vi "rszvl_core_global.vi"() -> ()   [LabVIEW 2014] (continued)
Repeated Capabilities"="", "Help"="This attribute returns the determined CREST factor (= ratio of peak power to average power) in dB.\n\nAvailable Repeated Capabilities:\nModifMinMaxAver: Min,Max,Aver\r\n\nRemote-control command(s):\nFETCh:BURSt:CRESt<[:AVERage] | :MAXimum|:MIMimum>?", "Flags"={"OPC Wait"=FALSE, "Dont check status"=FALSE, "*WAI"=FALSE}, "Check Status Callback"=""}, {"Level"=3, "Descriptive Name"="WLAN Fetch Rise Time", "Class Only"=FALSE, "Data Type"=1, "Access"=0, "Identifier"="RSZVL_ATTR_WLAN_FETC_TRIS", "Range Table"="", "Command"="FETC:BURS:TRIS:{ModifMinMaxAver}?", "Read Callback"="", "Write Callback"="", "Range Callback"="", "Check Callback"="", "Rngtable Callback"="", "Coerce Callback"="", "User Callback"="", "Supported Models"="", "Instrument Options"="", "Repeated Capabilities"="", "Restricted Repeated Capabilities"="", "Help"="This attribute returns the burst rise time in seconds.\n\nNote:\n(1) This attribute is valid only if standard IEEE 802.11b is selected.\n\nAvailable Repeated Capabilities:\nModifMinMaxAver: Min,Max,Aver\r\n\nRemote-control command(s):\nFETCh:BURSt:TRISe:<AVERage | MAXimum | MIMimum>?", "Flags"={"OPC Wait"=FALSE, "Dont check status"=FALSE, "*WAI"=FALSE}, "Check Status Callback"=""}, {"Level"=3, "Descriptive Name"="WLAN Fetch Fall Time", "Class Only"=FALSE, "Data Type"=1, "Access"=0, "Identifier"="RSZVL_ATTR_WLAN_FETC_TFAL", "Range Table"="", "Command"="FETC:BURS:TFAL:{ModifMinMaxAver}?", "Read Callback"="", "Write Callback"="", "Range Callback"="", "Check Callback"="", "Rngtable Callback"="", "Coerce Callback"="", "User Callback"="", "Supported Models"="", "Instrument Options"="", "Repeated Capabilities"="", "Restricted Repeated Capabilities"="", "Help"="This attribute returns the burst fall time in seconds.\n\nNote :\n(1) This attribute is available only for IEEE 802.11b standard.\n\nAvailable Repeated Capabilities:\nModifMinMaxAver: Min,Max,Aver\r\n\nRemote-control command(s):\nFETCh:BURSt:TFALl:<AVERage | MAXimum | MIMimum>?", "Flags"={"OPC Wait"=FALSE, "Dont check status"=FALSE, "*WAI"=FALSE}, "Check Status Callback"=""}, {"Level"=3, "Descriptive Name"="WLAN Fetch Frequency Error", "Class Only"=FALSE, "Data Type"=1, "Access"=0, "Identifier"="RSZVL_ATTR_WLAN_FETC_FERR", "Range Table"="", "Command"="FETC:BURS:FERR:{ModifMinMaxAver}?", "Read Callback"="", "Write Callback"="", "Range Callback"="", "Check Callback"="", "Rngtable Callback"="", "Coerce Callback"="", "User Callback"="", "Supported Models"="", "Instrument Options"="", "Repeated Capabilities"="", "Restricted Repeated Capabilities"="", "Help"="This attribute returns the measured frequency error in Hz.\n\nAvailable Repeated Capabilities:\nModifMinMaxAver: Min,Max,Aver\r\n\nRemote-control command(s):\nFETCh:BURSt:FERRor:<AVERage | MAXimum | MIMimum>?", "Flags"={"OPC Wait"=FALSE, "Dont check status"=FALSE, "*WAI"=FALSE}, "Check Status Callback"=""}, {"Level"=3, "Descriptive Name"="WLAN Fetch Symbol Error", "Class Only"=FALSE, "Data Type"=1, "Access"=0, "Identifier"="RSZVL_ATTR_WLAN_FETC_SYMB", "Range Table"="", "Command"="FETC:BURS:SYMB:{ModifMinMaxAver}?", "Read Callback"="", "Write Callback"="", "Range Callback"="", "Check Callback"="", "Rngtable Callback"="", "Coerce Callback"="", "User Callback"="", "Supported Models"="", "Instrument Options"="", "Repeated Capabilities"="", "Restricted Repeated Capabilities"="", "Help"="This attribute returns the number of symbols  that were outside the permissible demodulation\nrange within a burst.\n\nAvailable Repeated Capabilities:\nModifMinMaxAver: Min,Max,Aver\r\n\nRemote-control command(s):\nFETCh:BURSt:SYMBolerror:<AVERage | MAXimum | MIMimum>?", "Flags"={"OPC Wait"=FALSE, "Dont check status"=FALSE, "*WAI"=FALSE}, "Check Status Callback"=""}, {"Level"=3, "Descriptive Name"="WLAN Fetch IQ Offset Error", "Class Only"=FALSE, "Data Type"=1, "Access"=0, "Identifier"="RSZVL_ATTR_WLAN_FETC_IQOF", "Range Table"="", "Command"="FETC:BURS:IQOF:{ModifMinMaxAver}?", "Read Callback"="", "Write Callback"="", "Range Callback"="", "Check Callback"="", "Rngtable Callback"="", "Coerce Callback"="", "User Callback"="", "Supported Models"="", "Instrument Options"="", "Repeated Capabilities"="", "Restricted Repeated Capabilities"="", "Help"="This attribute returns the measured IQ offset errors in dB.\n\nAvailable Repeated Capabilities:\nModifMinMaxAver: Min,Max,Aver\r\n\nRemote-control command(s):\nFETCh:BURSt:IQOFfset:<AVERage | MAXimum | MIMimum>?", "Flags"={"OPC Wait"=FALSE, "Dont check status"=FALSE, "*WAI"=FALSE}, "Check Status Callback"=""}, {"Level"=3, "Descriptive Name"="WLAN Fetch IQ Imbalance Error", "Class Only"=FALSE, "Data Type"=1, "Access"=0, "Identifier"="RSZVL_ATTR_WLAN_FETC_GIMB", "Range Table"="", "Command"="FETC:BURS:GIMB:{ModifMinMaxAver}?", "Read Callback"="", "Write Callback"="", "Range Callback"="", "Check Callback"="", "Rngtable Callback"="", "Coerce Callback"="", "User Callback"="", "Supported Models"="", "Instrument Options"="", "Repeated Capabilities"="", "Restricted Repeated Capabilities"="", "Help"="This attribute returns the measured IQ imbalance errors in dB.\n\nAvailable Repeated Capabilities:\nModifMinMaxAver: Min,Max,Aver\r\n\nRemote-control command(s):\nFETCh:BURSt:GIMBalance:<AVERage | MAXimum | MIMimum>?", "Flags"={"OPC Wait"=FALSE, "Dont check status"=FALSE, "*WAI"=FALSE}, "Check Status Callback"=""}, {"Level"=3, "Descriptive Name"="WLAN Fetch Quadrature Error", "Class Only"=FALSE, "Data Type"=1, "Access"=0, "Identifier"="RSZVL_ATTR_WLAN_FETC_QUAD", "Range Table"="", "Command"="FETC:BURS:QUAD:{ModifMinMaxAver}?", "Read Callback"="", "Write Callback"="", "Range Callback"="", "Check Callback"="", "Rngtable Callback"="", "Coerce Callback"="", "User Callback"="", "Supported Models"="", "Instrument Options"="", "Repeated Capabilities"="", "Restricted Repeated Capabilities"="", "Help"="This attribute returns the accuracy in terms of the phase error of symbols within a burst.\nIt returns the angle error recorded for a symbol during the measurement.\n\nAvailable Repeated Capabilities:\nModifMinMaxAver: Min,Max,Aver\r\n\nRemote-control command(s):\nFETCh:BURSt:QUADoffset:<AVERage | MAXimum | MIMimum>?", "Flags"={"OPC Wait"=FALSE, "Dont check status"=FALSE, "*WAI"=FALSE}, "Check Status Callback"=""}, {"Level"=3, "Descriptive Name"="WLAN Fetch EVM", "Class Only"=FALSE, "Data Type"=1, "Access"=0, "Identifier"="RSZVL_ATTR_WLAN_FETC_EVM", "Range Table"="", "Command"="FETC:BURS:EVM:{ModifMinMaxAver}?", "Read Callback"="", "Write Callback"="", "Range Callback"="", "Check Callback"="", "Rngtable Callback"="", "Coerce Callback"="", "User Callback"="", "Supported Models"="", "Instrument Options"="", "Repeated Capabilities"="", "Restricted Repeated Capabilities"="", "Help"="This attribute returns the error vector magnitude measurement results summary in dB for the IEEE 802.11b standard. This result is the value before filtering.\n\nNote :\n(1) This attribute is available only for IEEE 802.11b standard.\n\nAvailable Repeated Capabilities:\nModifMinMaxAver: Min,Max,Aver\r\n\nRemote-control command(s):\nFETCh:BURSt:EVM:[IEEE]:<AVERage | MAXimum | MIMimum>?", "Flags"={"OPC Wait"=FALSE, "Dont check status"=FALSE, "*WAI"=FALSE}, "Check Status Callback"=""}, {"Level"=3, "Descriptive Name"="WLAN Fetch Filtered EVM", "Class Only"=FALSE, "Data Type"=1, "Access"=0, "Identifier"="RSZVL_ATTR_WLAN_FETC_EVM_DIR", "Range Table"="", "Command"="FETC:BURS:EVM:DIR:{ModifMinMaxAver}?", "Read Callback"="", "Write Callback"="", "Range Callback"="", "Check Callback"="", "Rngtable Callback"="", "Coerce Callback"="", "User Callback"="", "Supported Models"="", "Instrument Options"="", "Repeated Capabilities"="", "Restricted Repeated Capabilities"="", "Help"="This attribute returns the error vector magnitude measurement results summary in dB for the IEEE 802.11b standard. This result is the value after filtering.\n\nNote :\n(1) This attribute is available only for IEEE 802.11b standard.\n\nAvailable Repeated Capabilities:\nModifMinMaxAver: Min,Max,Aver\r\n\nRemote-control command(s):\nFETCh:BURSt:EVM:DIRect:<AVERage | MAXimum | MIMimum>?", "Flags"={"OPC Wait"=FALSE, "Dont check status"=FALSE, "*WAI"=FALSE}, "Check Status Callback"=""}, {"Level"=3, "Descriptive Name"="WLAN Fetch EVM All Carriers", "Class Only"=FALSE, "Data Type"=1, "Access"=0, "Identifier"="RSZVL_ATTR_WLAN_FETC_EVM_ALL", "Range Table"="", "Command"="FETC:BURS:EVM:ALL:{ModifMinMaxAver}?", "Read Callback"="", "Write Callback"="", "Range Callback"="", "Check Callback"="", "Rngtable Callback"="", "Coerce Callback"="", "User Callback"="", "Supported Models"="", "Instrument Options"="", "Repeated Capabilities"="", "Restricted Repeated Capabilities"="", "Help"="This attribute returns the error vector magnitude measurement results summary in dB. This is a combined figure that represents the pilot, data and the free carrier.\n\nAvailable Repeated Capabilities:\nModifMinMaxAver: Min,Max,Aver\r\n\nRemote-control command(s):\nFETCh:BURSt:EVM:ALL:<AVERage | MAXimum | MIMimum>?", "Flags"={"OPC Wait"=FALSE, "Dont check status"=FALSE, "*WAI"=FALSE}, "Check Status Callback"=""}, {"Level"=3, "Descriptive Name"="WLAN Fetch EVM Data Carriers", "Class Only"=FALSE, "Data Type"=1, "Access"=0, "Identifier"="RSZVL_ATTR_WLAN_FETC_EVM_DATA", "Range Table"="", "Command"="FETC:BURS:EVM:DATA:{ModifMinMaxAver}?", "Read Callback"="", "Write Callback"="", "Range Callback"="", "Check Callback"="", "Rngtable Callback"="", "Coerce Callback"="", "User Callback"="", "Supported Models"="", "Instrument Options"="", "Repeated Capabilities"="", "Restricted Repeated Capabilities"="", "Help"="This attribute returns the error vector magnitude measurement results summary for the data carrier\nin dB.\n\nAvailable Repeated Capabilities:\nModifMinMaxAver: Min,Max,Aver\r\n\nRemote-control command(s):\nFETCh:BURSt:EVM:DATA:<AVERage | MAXimum | MIMimum>?", "Flags"={"OPC Wait"=FALSE, "Dont check status"=FALSE, "*WAI"=FALSE}, "Check Status Callback"=""}, {"Level"=3, "Descriptive Name"="WLAN Fetch EVM Pilot Carriers", "Class Only"=FALSE, "Data Type"=1, "Access"=0, "Identifier"="RSZVL_ATTR_WLAN_FETC_EVM_PILOT", "Range Table"="", "Command"="FETC:BURS:EVM:PIL:{ModifMinMaxAver}?", "Read Callback"="", "Write Callback"="", "Range Callback"="", "Check Callback"="", "Rngtable Callback"="", "Coerce Callback"="", "User Callback"="", "Supported Models"="", "Instrument Options"="", "Repeated Capabilities"="", "Restricted Repeated Capabilities"="", "Help"="This attribute returns the error vector magnitude measurement results summary for the EVM pilot\ncarrier in dB.\n\nAvailable Repeated Capabilities:\nModifMinMaxAver: Min,Max,Aver\r\n\nRemote-control command(s):\nFETCh:BURSt:EVM:PILot:<AVERage | MAXimum | MIMimum>?", "Flags"={"OPC Wait"=FALSE, "Dont check status"=FALSE, "*WAI"=FALSE}, "Check Status Callback"=""}, {"Level"=3, "Descriptive Name"="WLAN Fetch Symbol Count", "Class Only"=FALSE, "Data Type"=0, "Access"=0, "Identifier"="RSZVL_ATTR_WLAN_FETC_SYMB_COUNT", "Range Table"="", "Command"="FETC:SYMB:COUNt?", "Read Callback"="", "Write Callback"="", "Range Callback"="", "Check Callback"="", "Rngtable Callback"="", "Coerce Callback"="", "User Callback"="", "Supported Models"="", "Instrument Options"="", "Repeated Capabilities"="", "Restricted Repeated Capabilities"="", "Help"="This attribute returns the number of symbols for each analyzed burst\n\nFW 3.70\n\nAvailable Repeated Capabilities:\nNone\n\nRemote-control command(s):\nFETCh:SYMBol:COUNt?", "Flags"={"OPC Wait"=FALSE, "Dont check status"=FALSE, "*WAI"=FALSE}, "Check Status Callback"=""}, {"Level"=2, "Descriptive Name"="Trigger Settings", "Class Only"=TRUE, "Data Type"=0, "Access"=0, "Identifier"="", "Range Table"="", "Command"="", "Read Callback"="", "Write Callback"="", "Range Callback"="", "Check Callback"="", "Rngtable Callback"="", "Coerce Callback"="", "User Callback"="", "Supported Models"="", "Instrument Options"="", "Repeated Capabilities"="", "Restricted Repeated Capabilities"="", "Help"="Attributes that configure the trigger.\n\n(1) WLAN Gate Delay Sample:\nThis attribute defines the gate delay in the capture buffer as a number of samples. The range of this value is dependent on the measurement that was last run.\n\n(2) WLAN Gate Delay Time:\nThis attribute defines the gate delay in the capture buffer in time units. The range of this value is\ndependent on the measurement that was last run.\n\n(3) WLAN Gate Length Sample:\nThis attribute defines the gate time in the capture buffer as a number of samples. The range of this\nvalue is dependent on the measurement that was last run.\n\n(4) WLAN Gate Length Time:\nThis attribute defines the gate time in the capture buffer in time units. The range of this value is\ndependent on the measurement that was last run.\n\n(5) WLAN Link Gate And Marker:\nThis attribute links together the movement of the gating lines and the capture buffer marker.\n\n(6) WLAN Gating:\nThis attribute switches the gating on/off .\n\n(7) WLAN Trigger Mode:\nThis attribute configures how triggering is to be performed.\n\n(8) WLAN Trigger Power Level:\nThis attribute accepts the level of the input signal for which triggering will occur. The value is\nspecified in dBm for RF input and V for baseband inputs.\n\n(9) WLAN Trigger Auto Level:\nThis attribute specifies whether or not an automatic power trigger level calculation is performed\nbefore each main measurement. The setting of this command is ignored if the setting for\nTRIGger[:SEQuence]:MODE is not POWer.", "Flags"={"OPC Wait"=FALSE, "Dont check status"=FALSE, "*WAI"=FALSE}, "Check Status Callback"=""}, {"Level"=3, "Descriptive Name"="WLAN Gate Delay Sample", "Class Only"=FALSE, "Data Type"=0, "Access"=2, "Identifier"="RSZVL_ATTR_WLAN_EGAT_HOLD_SAMP", "Range Table"="", "Command"="SWE:EGAT:HOLD:SAMP", "Read Callback"="", "Write Callback"="", "Range Callback"="", "Check Callback"="", "Rngtable Callback"="", "Coerce Callback"="", "User Callback"="", "Supported Models"="", "Instrument Options"="", "Repeated Capabilities"="", "Restricted Repeated Capabilities"="", "Help"="This attribute defines the gate delay in the capture buffer as a number of samples. The range of this value is dependent on the measurement that was last run.\n\nAvailable Repeated Capabilities:\nNone\n\nRemote-control command(s):\n[SENSe:]SWEep:EGATe:HOLDoff:SAMPle", "Flags"={"OPC Wait"=FALSE, "Dont check status"=FALSE, "*WAI"=FALSE}, "Check Status Callback"=""}, {"Level"=3, "Descriptive Name"="WLAN Gate Delay Time", "Class Only"=FALSE, "Data Type"=1, "Access"=2, "Identifier"="RSZVL_ATTR_WLAN_EGAT_HOLD_TIME", "Range Table"="", "Command"="SWE:EGAT:HOLD", "Read Callback"="", "Write Callback"="", "Range Callback"="", "Check Callback"="", "Rngtable Callback"="", "Coerce Callback"="", "User Callback"="", "Supported Models"="", "Instrument Options"="", "Repeated Capabilities"="", "Restricted Repeated Capabilities"="", "Help"="This attribute defines the gate delay in the capture buffer in time units. The range of this value is\ndependent on the measurement that was last run.\n\nAvailable Repeated Capabilities:\nNone\n\nRemote-control command(s):\n[SENSe:]SWEep:EGATe:HOLDoff[:TIMe]", "Flags"={"OPC Wait"=FALSE, "Dont check status"=FALSE, "*WAI"=FALSE}, "Check Status Callback"=""}, {"Level"=3, "Descriptive Name"="WLAN Gate Length Sample", "Class Only"=FALSE, "Data Type"=0, "Access"=2, "Identifier"="RSZVL_ATTR_WLAN_EGAT_LENG_SAMP", "Range Table"="", "Command"="SWE:EGAT:LENG:SAMP", "Read Callback"="", "Write Callback"="", "Range Callback"="", "Check Callback"="", "Rngtable Callback"="", "Coerce Callback"="", "User Callback"="", "Supported Models"="", "Instrument Options"="", "Repeated Capabilities"="", "Restricted Repeated Capabilities"="", "Help"="This attribute defines the gate time in the capture buffer as a number of samples. The range of this\nvalue is dependent on the measurement that was last run.\n\nAvailable Repeated Capabilities:\nNone\n\nRemote-control command(s):\n[SENSe:]SWEep:EGATe:LENGth:SAMPle", "Flags"={"OPC Wait"=FALSE, "Dont check status"=FALSE, "*WAI"=FALSE}, "Check Status Callback"=""}, {"Level"=3, "Descriptive Name"="WLAN Gate Length Time", "Class Only"=FALSE, "Data Type"=1, "Access"=2, "Identifier"="RSZVL_ATTR_WLAN_EGAT_LENG_TIME", "Range Table"="", "Command"="SWE:EGAT:LENG", "Read Callback"="", "Write Callback"="", "Range Callback"="", "Check Callback"="", "Rngtable Callback"="", "Coerce Callback"="", "User Callback"="", "Supported Models"="", "Instrument Options"="", "Repeated Capabilities"="", "Restricted Repeated Capabilities"="", "Help"="This attribute defines the gate time in the capture buffer in time units. The range of this value is\ndependent on the measurement that was last run.\n\nAvailable Repeated Capabilities:\nNone\n\nRemote-control command(s):\n[SENSe:]SWEep:EGATe:LENGth[:TIMe]", "Flags"={"OPC Wait"=FALSE, "Dont check status"=FALSE, "*WAI"=FALSE}, "Check Status Callback"=""}, {"Level"=3, "Descriptive Name"="WLAN Link Gate And Marker", "Class Only"=FALSE, "Data Type"=3, "Access"=2, "Identifier"="RSZVL_ATTR_WLAN_EGAT_LINK", "Range Table"="", "Command"="SWE:EGAT:LINK", "Read Callback"="", "Write Callback"="", "Range Callback"="", "Check Callback"="", "Rngtable Callback"="", "Coerce Callback"="", "User Callback"="", "Supported Models"="", "Instrument Options"="", "Repeated Capabilities"="", "Restricted Repeated Capabilities"="", "Help"="This attribute links together the movement of the gating lines and the capture buffer marker.\n\nAvailable Repeated Capabilities:\nNone\n\nRemote-control command(s):\n[SENSe:]SWEep:EGATe:LINK ON | OFF", "Flags"={"OPC Wait"=FALSE, "Dont check status"=FALSE, "*WAI"=FALSE}, "Check Status Callback"=""}, {"Level"=3, "Descriptive Name"="WLAN Gating", "Class Only"=FALSE, "Data Type"=3, "Access"=2, "Identifier"="RSZVL_ATTR_WLAN_EGAT", "Range Table"="", "Command"="SWE:EGAT", "Read Callback"="", "Write Callback"="", "Range Callback"="", "Check Callback"="", "Rngtable Callback"="", "Coerce Callback"="", "User Callback"="", "Supported Models"="", "Instrument Options"="", "Repeated Capabilities"="", "Restricted Repeated Capabilities"="", "Help"="This attribute switches the gating on/off .\n\nAvailable Repeated Capabilities:\nNone\n\nRemote-control command(s):\n[SENSe:]SWEep:EGATe ON | OFF", "Flags"={"OPC Wait"=FALSE, "Dont check status"=FALSE, "*WAI"=FALSE}, "Check Status Callback"=""}, {"Level"=3, "Descriptive Name"="WLAN Trigger Mode", "Class Only"=FALSE, "Data Type"=0, "Access"=2, "Identifier"="RSZVL_ATTR_WLAN_TRIG_MODE", "Range Table"="rszvl_rngTrigMode", "Command"="TRIG:MODE", "Read Callback"="", "Write Callback"="", "Range Callback"="", "Check Callback"="", "Rngtable Callback"="", "Coerce Callback"="", "User Callback"="", "Supported Models"="", "Instrument Options"="", "Repeated Capabilities"="", "Restricted Repeated Capabilities"="", "Help"="This attribute configures how triggering is to be performed.\n\nAvailable Repeated Capabilities:\nNone\n\nRemote-control command(s):\nTRIGger[:SEQuence]:MODE IMMediate | EXTernal | POWer", "Flags"={"OPC Wait"=FALSE, "Dont check status"=FALSE, "*WAI"=FALSE}, "Check Status Callback"=""}, {"Level"=3, "Descriptive Name"="WLAN Trigger Power Level", "Class Only"=FALSE, "Data Type"=1, "Access"=2, "Identifier"="RSZVL_ATTR_WLAN_TRIG_POW_LEV", "Range Table"="", "Command"="TRIG:LEV:POW", "Read Callback"="", "Write Callback"="", "Range Callback"="", "Check Callback"="", "Rngtable Callback"="", "Coerce Callback"="", "User Callback"="", "Supported Models"="", "Instrument Options"="", "Repeated Capabilities"="", "Restricted Repeated Capabilities"="", "Help"="This attribute accepts the level of the input signal for which triggering will occur. The value is\nspecified in dBm for RF input and V for baseband inputs.\n\nAvailable Repeated Capabilities:\nNone\n\nRemote-control command(s):\nTRIGger[:SEQuence]:LEVel:POWer", "Flags"={"OPC Wait"=FALSE, "Dont check status"=FALSE, "*WAI"=FALSE}, "Check Status Callback"=""}, {"Level"=3, "Descriptive Name"="WLAN Trigger Auto Level", "Class Only"=FALSE, "Data Type"=3, "Access"=2, "Identifier"="RSZVL_ATTR_WLAN_TRIG_POW_LEV_AUTO", "Range Table"="", "Command"="TRIG:LEV:POW:AUTO", "Read Callback"="", "Write Callback"="", "Range Callback"="", "Check Callback"="", "Rngtable Callback"="", "Coerce Callback"="", "User Callback"="", "Supported Models"="", "Instrument Options"="", "Repeated Capabilities"="", "Restricted Repeated Capabilities"="", "Help"="This attribute specifies whether or not an automatic power trigger level calculation is performed\nbefore each main measurement. The setting of this command is ignored if the setting for\nTRIGger[:SEQuence]:MODE is not POWer.\n\nAvailable Repeated Capabilities:\nNone\n\nRemote-control command(s):\nTRIGger[:SEQuence]:LEVel:POWer:AUTO", "Flags"={"OPC Wait"=FALSE, "Dont check status"=FALSE, "*WAI"=FALSE}, "Check Status Callback"=""}, {"Level"=2, "Descriptive Name"="Demodulation Settings", "Class Only"=TRUE, "Data Type"=0, "Access"=0, "Identifier"="", "Range Table"="", "Command"="", "Read Callback"="", "Write Callback"="", "Range Callback"="", "Check Callback"="", "Rngtable Callback"="", "Coerce Callback"="", "User Callback"="", "Supported Models"="", "Instrument Options"="", "Repeated Capabilities"="", "Restricted Repeated Capabilities"="", "Help"="Attributes that configure the demodulation.\n\n(1) WLAN Channel Estimation:\nThis attribute defines whether channel estimation will be done in the preamble and payload (if set\nto 1) or only in the preamble (if set to 0). The effect of this is most noticeable for the EVM\nmeasurement results, where the results will be improved when this feature is enabled.\nHowever, this functionality is not supported by the IEEE 802.11a standard and must be disabled if the\nresults are to be strictly measured against the standard.\n\n(2) WLAN Use Signal Field Content:\nThis attribute sets the signal symbol field. If is set to ON, the signal symbol field of the burst is analyzed to determine the details of the burst. When this field is set to ON, only bursts that match the supplied burst type and modulation are considered in results analysis. \n\nNote:\n(1) For IEEE 802.11b, this attribute sets PLCP Header Content.\n\n(3) WLAN Auto Demodulation:\nThis attribute sets the burst to analyze auto demodulation state. is set to ON, the signal symbol field of the burst is analyzed to determine the\nmodulation scheme of the first burst. When this field is set to ON, only bursts that match the\nmodulation scheme are considered in results analysis.\n\nNote:\n(1) This attribute is available only if Signal field content is set ON.\n\n(4) WLAN Demodulator:\nThis attribute sets the analysis modulation format that will be assumed when the measurement is performed. If the [SENSe:]DEMod:FORMat:SIGSymbol parametrer has been set to ON, this command can be used to measure only certain burst types within a measurement sequence.\n\nValues:\nFor IEEE 802.11b & g (Single Carrier) standard:\nRSZVL_VAL_WLAN_DBPSK,\nRSZVL_VAL_WLAN_DQPSK,\nRSZVL_VAL_WLAN_CCK55\nRSZVL_VAL_WLAN_CCK11\nRSZVL_VAL_WLAN_PBCC55\nRSZVL_VAL_WLAN_PBCC11\nRSZVL_VAL_WLAN_PBCC22\n\nDBPSK - Differential BI-Phase shift keying\nDQPSK - Differential Quadrature phase shift keying\nCCK55 - Complementary Code Keying at 5.5 Mbps\nCCK11 - Complementary Code Keying at 11 Mbps\nPBCC55 - PBCC at 5.5 Mbps\nPBCC11 - PBCC at 11 Mbps\nPBCC22 - PBCC at 11 Mbps\n\nFor standard IEEE 802.11j (10 MHz): \nRSZVL_VAL_WLAN_BPSK3,\nRSZVL_VAL_WLAN_BPSK45,\nRSZVL_VAL_WLAN_QPSK6,\nRSZVL_VAL_WLAN_QPSK9,\nRSZVL_VAL_WLAN_QAM1612,\nRSZVL_VAL_WLAN_QAM1618,\nRSZVL_VAL_WLAN_QAM6424,\nRSZVL_VAL_WLAN_QAM6427,\n\nBPSK3 - BI-Phase shift keying at 3 Mbps\nBPSK45 - BI-Phase shift keying at 6 Mbps\nQPSK6 - Quadrature phase shift keying at 6 Mbps\nQPSK9 - Quadrature phase shift keying at 9 Mbps\nQAM1612 - Quadrature Amplitude Modulation at 12 Mbps\nQAM1618 - Quadrature Amplitude Modulation at 18 Mbps\nQAM6424 - Quadrature Amplitude Modulation at 24 Mbps\nQAM6427 - Quadrature Amplitude Modulation at 27 Mbps\n\nFor standard IEEE 802.11a, g (OFDM), j (20 MHz):\nRSZVL_VAL_WLAN_BPSK6,\nRSZVL_VAL_WLAN_BPSK9,\nRSZVL_VAL_WLAN_QPSK12,\nRSZVL_VAL_WLAN_QPSK18,\nRSZVL_VAL_WLAN_QAM1624,\nRSZVL_VAL_WLAN_QAM1636,\nRSZVL_VAL_WLAN_QAM6448,\nRSZVL_VAL_WLAN_QAM6454,\n\nBPSK6 - BI-Phase shift keying at 6 Mbps\nBPSK9 - BI-Phase shift keying at 9 Mbps\nQPSK12 - Quadrature phase shift keying at 12 Mbps\nQPSK18 - Quadrature phase shift keying at 18 Mbps\nQAM1624 - Quadrature Amplitude Modulation at 24 Mbps\nQAM1636 - Quadrature Amplitude Modulation at 36 Mbps\nQAM6448 - Quadrature Amplitude Modulation at 48 Mbps\nQAM6454 - Quadrature Amplitude Modulation at 54 Mbps\n\nfor WiMAX:\nRSZVL_VAL_WLAN_BPSK1_2,\nRSZVL_VAL_WLAN_QPSK1_2,\nRSZVL_VAL_WLAN_QPSK3_4,\nRSZVL_VAL_WLAN_16QAM1_2,\nRSZVL_VAL_WLAN_16QAM3_4,\nRSZVL_VAL_WLAN_64QAM2_3\n\nBPSK1/2\nQPSK1/2\nQPSK3/4\n16QAM1/2\n16QAM3/4\n64QAM2/3\n\n\n(5) WLAN Equal Burst Length:\nThis attribute enables/disables equal burst length to analyze. When this attribute is set to ON, only bursts of equal length will take part in the measurement analysis. In this case, the value specified with \n[SENSe:]DEMod:FORMat:BANalyze:SYMbols:MIN command sets the number of symbols that a burst must have in order to take part in analysis\n\nNote:\n(1) This attribute is not valid for IEEE 802.11b standard.\n\n(6) WLAN Number of Data Symbols:\nThis attribute specifies the number of data symbols required for bursts to qualify for measurement\nanalysis. Only bursts with the specified number of symbols will be used in the measurement analysis. The number of data symbols is defined as the uncoded bits including service and tail bits.\n\nNote:\n(1) This attribute is not valid for IEEE 802.11b standard.\n\n(7) WLAN Equal Burst Length in Bytes:\nThis attribute defines, if bursts of equal length will take part in the measurement analysis.\nWhen this command is set to true, the value specified by the [SENSe:]DEMod:FORMat:\nBANalyze:DBYTes:MIN command specifies the number of data bytes that a burst must have in order to take part in measurement analysis.\n\nNote:\n(1) This attribute is valid only for IEEE 802.11b standard.\n\n(8) WLAN Payload Length in Bytes:\nThis attribute specifies the number of data bytes required for bursts to qualify for measurement\nanalysis. Only bursts with the specified number of data bytes will be used in the measurement analysis. When the  [SENSe:]DEMod:FORMat:BANalyze:DBYTes:EQUal command has been set to true, this command specifies the exact number of data bytes required for a burst to take part in measurement analysis. When the [SENSe:]DEMod:BANalyze:DBYTes:EQUal command is set to false, this command specifies the minimum number of data bytes required for a burst to take part in measurement analysis.\n\nNote:\n(1) This attribute is valid only for IEEE 802.11b standard.\n\n(9) WLAN Equal Burst Length in Time:\nThis attribute defines, if only bursts of equal length will take part in the PVT analysis.\nWhen this command is set to true, the value specified by the\n[SENSe:]DEMod:BANalyze:DURation:MIN command specifies the required burst duration in order\nfor a burst to take part in measurement analysis.\n\nNote:\n(1) This attribute is valid only for IEEE 802.11b/g standard.\n\n(10) WLAN Payload Length in Time:\nThis attribute specifies the duration in microseconds required for bursts to qualify for measurement analysis. Only bursts with the specified duration will be used in the measurement analysis. When the \n[SENSe:]DEMod:BANalyze:DURation:EQUal command has been set to true, this command specifies the exact duration required for a burst to take part in measurement analysis. When the [SENSe:]DEMod:BANalyze:DBYTes:EQUal command is set to false, this command specifies the minimum duration required for a burst to take part in measurement analysis.\n\nNote:\n(1) This attribute is valid only for IEEE 802.11b/g standard.\n\n(11) WLAN Tracking Level:\nThis attribute defines whether or not the measurement results should be compensated for level.\n\n(12) WLAN Tracking Phase:\nThis attribute defines whether or not the measurement results should be compensated for phase.\n\n(13) WLAN Tracking Timing:\nThis attribute defines whether or not the measurement results should be compensated for time.", "Flags"={"OPC Wait"=FALSE, "Dont check status"=FALSE, "*WAI"=FALSE}, "Check Status Callback"=""}, {"Level"=3, "Descriptive Name"="WLAN Channel Estimation", "Class Only"=FALSE, "Data Type"=3, "Access"=2, "Identifier"="RSZVL_ATTR_WLAN_CEST", "Range Table"="", "Command"="DEM:CEST", "Read Callback"="", "Write Callback"="", "Range Callback"="", "Check Callback"="", "Rngtable Callback"="", "Coerce Callback"="", "User Callback"="", "Supported Models"="", "Instrument Options"="", "Repeated Capabilities"="", "Restricted Repeated Capabilities"="", "Help"="This attribute defines whether channel estimation will be done in the preamble and payload (if set\nto 1) or only in the preamble (if set to 0). The effect of this is most noticeable for the EVM\nmeasurement results, where the results will be improved when this feature is enabled.\nHowever, this functionality is not supported by the IEEE 802.11a standard and must be disabled if the\nresults are to be strictly measured against the standard.\n\nAvailable Repeated Capabilities:\nNone\n\nRemote-control command(s):\n[SENSe:]DEMod:CESTimation", "Flags"={"OPC Wait"=FALSE, "Dont check status"=FALSE, "*WAI"=FALSE}, "Check Status Callback"=""}, {"Level"=3, "Descriptive Name"="WLAN Use Signal Field Content", "Class Only"=FALSE, "Data Type"=3, "Access"=2, "Identifier"="RSZVL_ATTR_WLAN_SIGS", "Range Table"="", "Command"="DEM:FORM:SIGS", "Read Callback"="", "Write Callback"="", "Range Callback"="", "Check Callback"="", "Rngtable Callback"="", "Coerce Callback"="", "User Callback"="", "Supported Models"="", "Instrument Options"="", "Repeated Capabilities"="", "Restricted Repeated Capabilities"="", "Help"="This attribute sets the signal symbol field. If is set to ON, the signal symbol field of the burst is analyzed to determine the details of the burst. When this field is set to ON, only bursts that match the supplied burst type and modulation are considered in results analysis. \n\nNote:\n(1) For IEEE 802.11b, this attribute sets PLCP Header Content.\n\nAvailable Repeated Capabilities:\nNone\n\nRemote-control command(s):\n[SENSe:]DEMod:FORMat:SIGSymbol ON | OFF", "Flags"={"OPC Wait"=FALSE, "Dont check status"=FALSE, "*WAI"=FALSE}, "Check Status Callback"=""}, {"Level"=3, "Descriptive Name"="WLAN Auto Demodulation", "Class Only"=FALSE, "Data Type"=3, "Access"=2, "Identifier"="RSZVL_ATTR_WLAN_BCON_AUTO", "Range Table"="", "Command"="DEM:FORM:AUTO", "Read Callback"="", "Write Callback"="", "Range Callback"="", "Check Callback"="", "Rngtable Callback"="", "Coerce Callback"="", "User Callback"="", "Supported Models"="", "Instrument Options"="", "Repeated Capabilities"="", "Restricted Repeated Capabilities"="", "Help"="This attribute sets the burst to analyze auto demodulation state. is set to ON, the signal symbol field of the burst is analyzed to determine the\nmodulation scheme of the first burst. When this field is set to ON, only bursts that match the\nmodulation scheme are considered in results analysis.\n\nNote:\n(1) This attribute is available only if Signal field content is set ON.\n\nAvailable Repeated Capabilities:\nNone\n\nRemote-control command(s):\n[SENSe:]DEMod:FORMat[:BCONtent]:AUTO ON | OFF", "Flags"={"OPC Wait"=FALSE, "Dont check status"=FALSE, "*WAI"=FALSE}, "Check Status Callback"=""}, {"Level"=3, "Descriptive Name"="WLAN Demodulator", "Class Only"=FALSE, "Data Type"=0, "Access"=2, "Identifier"="RSZVL_ATTR_WLAN_BAN", "Range Table"="rszvl_rngWlanDemod", "Command"="DEM:FORM:BAN", "Read Callback"="", "Write Callback"="rszvl_burstType_WriteCallback.vi", "Range Callback"="", "Check Callback"="", "Rngtable Callback"="", "Coerce Callback"="", "User Callback"="", "Supported Models"="", "Instrument Options"="", "Repeated Capabilities"="", "Restricted Repeated Capabilities"="", "Help"="This attribute sets the analysis modulation format that will be assumed when the measurement is performed. If the [SENSe:]DEMod:FORMat:SIGSymbol parametrer has been set to ON, this command can be used to measure only certain burst types within a measurement sequence.\n\nValues:\nFor IEEE 802.11b & g (Single Carrier) standard:\nRSZVL_VAL_WLAN_DBPSK,\nRSZVL_VAL_WLAN_DQPSK,\nRSZVL_VAL_WLAN_CCK55\nRSZVL_VAL_WLAN_CCK11\nRSZVL_VAL_WLAN_PBCC55\nRSZVL_VAL_WLAN_PBCC11\nRSZVL_VAL_WLAN_PBCC22\n\nDBPSK - Differential BI-Phase shift keying\nDQPSK - Differential Quadrature phase shift keying\nCCK55 - Complementary Code Keying at 5.5 Mbps\nCCK11 - Complementary Code Keying at 11 Mbps\nPBCC55 - PBCC at 5.5 Mbps\nPBCC11 - PBCC at 11 Mbps\nPBCC22 - PBCC at 11 Mbps\n\nFor standard IEEE 802.11j (10 MHz): \nRSZVL_VAL_WLAN_BPSK3,\nRSZVL_VAL_WLAN_BPSK45,\nRSZVL_VAL_WLAN_QPSK6,\nRSZVL_VAL_WLAN_QPSK9,\nRSZVL_VAL_WLAN_QAM1612,\nRSZVL_VAL_WLAN_QAM1618,\nRSZVL_VAL_WLAN_QAM6424,\nRSZVL_VAL_WLAN_QAM6427,\n\nBPSK3 - BI-Phase shift keying at 3 Mbps\nBPSK45 - BI-Phase shift keying at 6 Mbps\nQPSK6 - Quadrature phase shift keying at 6 Mbps\nQPSK9 - Quadrature phase shift keying at 9 Mbps\nQAM1612 - Quadrature Amplitude Modulation at 12 Mbps\nQAM1618 - Quadrature Amplitude Modulation at 18 Mbps\nQAM6424 - Quadrature Amplitude Modulation at 24 Mbps\nQAM6427 - Quadrature Amplitude Modulation at 27 Mbps\n\nFor standard IEEE 802.11a, g (OFDM), j (20 MHz):\nRSZVL_VAL_WLAN_BPSK6,\nRSZVL_VAL_WLAN_BPSK9,\nRSZVL_VAL_WLAN_QPSK12,\nRSZVL_VAL_WLAN_QPSK18,\nRSZVL_VAL_WLAN_QAM1624,\nRSZVL_VAL_WLAN_QAM1636,\nRSZVL_VAL_WLAN_QAM6448,\nRSZVL_VAL_WLAN_QAM6454,\n\nBPSK6 - BI-Phase shift keying at 6 Mbps\nBPSK9 - BI-Phase shift keying at 9 Mbps\nQPSK12 - Quadrature phase shift keying at 12 Mbps\nQPSK18 - Quadrature phase shift keying at 18 Mbps\nQAM1624 - Quadrature Amplitude Modulation at 24 Mbps\nQAM1636 - Quadrature Amplitude Modulation at 36 Mbps\nQAM6448 - Quadrature Amplitude Modulation at 48 Mbps\nQAM6454 - Quadrature Amplitude Modulation at 54 Mbps\n\nfor WiMAX:\nRSZVL_VAL_WLAN_BPSK1_2,\nRSZVL_VAL_WLAN_QPSK1_2,\nRSZVL_VAL_WLAN_QPSK3_4,\nRSZVL_VAL_WLAN_16QAM1_2,\nRSZVL_VAL_WLAN_16QAM3_4,\nRSZVL_VAL_WLAN_64QAM2_3\n\nBPSK1/2\nQPSK1/2\nQPSK3/4\n16QAM1/2\n16QAM3/4\n64QAM2/3\n\nAvailable Repeated Capabilities:\nNone\n\nRemote-control command(s):\n[SENSe:]DEMod:FORMat:BANalyze", "Flags"={"OPC Wait"=FALSE, "Dont check status"=FALSE, "*WAI"=FALSE}, "Check Status Callback"=""}, {"Level"=3, "Descriptive Name"="WLAN Equal Burst Length", "Class Only"=FALSE, "Data Type"=3, "Access"=2, "Identifier"="RSZVL_ATTR_WLAN_SYM_EQU", "Range Table"="", "Command"="DEM:FORM:BAN:SYMB:EQU", "Read Callback"="", "Write Callback"="", "Range Callback"="", "Check Callback"="", "Rngtable Callback"="", "Coerce Callback"="", "User Callback"="", "Supported Models"="", "Instrument Options"="", "Repeated Capabilities"="", "Restricted Repeated Capabilities"="", "Help"="This attribute enables/disables equal burst length to analyze. When this attribute is set to ON, only bursts of equal length will take part in the measurement analysis. In this case, the value specified with \n[SENSe:]DEMod:FORMat:BANalyze:SYMbols:MIN command sets the number of symbols that a burst must have in order to take part in analysis\n\nNote:\n(1) This attribute is not valid for IEEE 802.11b standard.\n\nAvailable Repeated Capabilities:\nNone\n\nRemote-control command(s):\n[SENSe:]DEMod:FORMat:BANalyze:SYMBols:EQUal ON | OFF", "Flags"={"OPC Wait"=FALSE, "Dont check status"=FALSE, "*WAI"=FALSE}, "Check Status Callback"=""}, {"Level"=3, "Descriptive Name"="WLAN Number of Data Symbols", "Class Only"=FALSE, "Data Type"=0, "Access"=2, "Identifier"="RSZVL_ATTR_WLAN_SYM", "Range Table"="", "Command"="DEM:FORM:BAN:SYMB:{ModifMinMaxAver}", "Read Callback"="", "Write Callback"="", "Range Callback"="", "Check Callback"="", "Rngtable Callback"="", "Coerce Callback"="", "User Callback"="", "Supported Models"="", "Instrument Options"="", "Repeated Capabilities"="", "Restricted Repeated Capabilities"="", "Help"="This attribute specifies the number of data symbols required for bursts to qualify for measurement\nanalysis. Only bursts with the specified number of symbols will be used in the measurement analysis. The number of data symbols is defined as the uncoded bits including service and tail bits.\n\nNote:\n(1) This attribute is not valid for IEEE 802.11b standard.\n\nAvailable Repeated Capabilities:\nModifMinMaxAver: Min,Max,Aver\r\n\nRemote-control command(s):\n[SENSe:]DEMod:FORMat:BANalyze:SYMBols:<MAX | MIN>", "Flags"={"OPC Wait"=FALSE, "Dont check status"=FALSE, "*WAI"=FALSE}, "Check Status Callback"=""}, {"Level"=3, "Descriptive Name"="WLAN Equal Burst Length in Bytes", "Class Only"=FALSE, "Data Type"=3, "Access"=2, "Identifier"="RSZVL_ATTR_WLAN_DBYT_EQU", "Range Table"="", "Command"="DEM:FORM:BAN:DBYT:EQU", "Read Callback"="", "Write Callback"="", "Range Callback"="", "Check Callback"="", "Rngtable Callback"="", "Coerce Callback"="", "User Callback"="", "Supported Models"="", "Instrument Options"="", "Repeated Capabilities"="", "Restricted Repeated Capabilities"="", "Help"="This attribute defines, if bursts of equal length will take part in the measurement analysis.\nWhen this command is set to true, the value specified by the [SENSe:]DEMod:FORMat:\nBANalyze:DBYTes:MIN command specifies the number of data bytes that a burst must have in order to take part in measurement analysis.\n\nNote:\n(1) This attribute is valid only for IEEE 802.11b standard.\n\nAvailable Repeated Capabilities:\nNone\n\nRemote-control command(s):\n[SENSe:]DEMod:FORMat:BANalyze:DBYTes:EQUal", "Flags"={"OPC Wait"=FALSE, "Dont check status"=FALSE, "*WAI"=FALSE}, "Check Status Callback"=""}, {"Level"=3, "Descriptive Name"="WLAN Payload Length in Bytes", "Class Only"=FALSE, "Data Type"=0, "Access"=2, "Identifier"="RSZVL_ATTR_WLAN_DBYT", "Range Table"="rszvl_rngWlanDbyte", "Command"="DEM:FORM:BAN:DBYT:{ModifMinMaxAver}", "Read Callback"="", "Write Callback"="", "Range Callback"="", "Check Callback"="", "Rngtable Callback"="", "Coerce Callback"="", "User Callback"="", "Supported Models"="", "Instrument Options"="", "Repeated Capabilities"="", "Restricted Repeated Capabilities"="", "Help"="This attribute specifies the number of data bytes required for bursts to qualify for measurement\nanalysis. Only bursts with the specified number of data bytes will be used in the measurement analysis. When the  [SENSe:]DEMod:FORMat:BANalyze:DBYTes:EQUal command has been set to true, this command specifies the exact number of data bytes required for a burst to take part in measurement analysis. When the [SENSe:]DEMod:BANalyze:DBYTes:EQUal command is set to false, this command specifies the minimum number of data bytes required for a burst to take part in measurement analysis.\n\nNote:\n(1) This attribute is valid only for IEEE 802.11b standard.\n\nAvailable Repeated Capabilities:\nModifMinMaxAver: Min,Max,Aver\r\n\nRemote-control command(s):\n[SENSe:]DEMod:FORMat:BANalyze:DBYTes:<MAX | MIN>", "Flags"={"OPC Wait"=FALSE, "Dont check status"=FALSE, "*WAI"=FALSE}, "Check Status Callback"=""}, {"Level"=3, "Descriptive Name"="WLAN Equal Burst Length in Time", "Class Only"=FALSE, "Data Type"=3, "Access"=2, "Identifier"="RSZVL_ATTR_WLAN_DUR_EQU", "Range Table"="", "Command"="DEM:FORM:BAN:DUR:EQU", "Read Callback"="", "Write Callback"="", "Range Callback"="", "Check Callback"="", "Rngtable Callback"="", "Coerce Callback"="", "User Callback"="", "Supported Models"="", "Instrument Options"="", "Repeated Capabilities"="", "Restricted Repeated Capabilities"="", "Help"="This attribute defines, if only bursts of equal length will take part in the PVT analysis.\nWhen this command is set to true, the value specified by the\n[SENSe:]DEMod:BANalyze:DURation:MIN command specifies the required burst duration in order\nfor a burst to take part in measurement analysis.\n\nNote:\n(1) This attribute is valid only for IEEE 802.11b/g standard.\n\nAvailable Repeated Capabilities:\nNone\n\nRemote-control command(s):\n[SENSe:]DEMod:FORMat:BANalyze:DURation:EQUal", "Flags"={"OPC Wait"=FALSE, "Dont check status"=FALSE, "*WAI"=FALSE}, "Check Status Callback"=""}, {"Level"=3, "Descriptive Name"="WLAN Payload Length in Time", "Class Only"=FALSE, "Data Type"=0, "Access"=2, "Identifier"="RSZVL_ATTR_WLAN_DUR", "Range Table"="", "Command"="DEM:FORM:BAN:DUR:{ModifMinMaxAver}", "Read Callback"="", "Write Callback"="", "Range Callback"="", "Check Callback"="", "Rngtable Callback"="", "Coerce Callback"="", "User Callback"="", "Supported Models"="", "Instrument Options"="", "Repeated Capabilities"="", "Restricted Repeated Capabilities"="", "Help"="This attribute specifies the duration in microseconds required for bursts to qualify for measurement analysis. Only bursts with the specified duration will be used in the measurement analysis. When the \n[SENSe:]DEMod:BANalyze:DURation:EQUal command has been set to true, this command specifies the exact duration required for a burst to take part in measurement analysis. When the [SENSe:]DEMod:BANalyze:DBYTes:EQUal command is set to false, this command specifies the minimum duration required for a burst to take part in measurement analysis.\n\nNote:\n(1) This attribute is valid only for IEEE 802.11b/g standard.\n\nAvailable Repeated Capabilities:\nModifMinMaxAver: Min,Max,Aver\r\n\nRemote-control command(s):\n[SENSe:]DEMod:FORMat:BANalyze:DURation:<MAX | MIN>", "Flags"={"OPC Wait"=FALSE, "Dont check status"=FALSE, "*WAI"=FALSE}, "Check Status Callback"=""}, {"Level"=3, "Descriptive Name"="WLAN Tracking Level", "Class Only"=FALSE, "Data Type"=3, "Access"=2, "Identifier"="RSZVL_ATTR_WLAN_TRAC_LEV", "Range Table"="", "Command"="SENS:TRAC:LEV", "Read Callback"="", "Write Callback"="", "Range Callback"="", "Check Callback"="", "Rngtable Callback"="", "Coerce Callback"="", "User Callback"="", "Supported Models"="", "Instrument Options"="", "Repeated Capabilities"="", "Restricted Repeated Capabilities"="", "Help"="This attribute defines whether or not the measurement results should be compensated for level.\n\nAvailable Repeated Capabilities:\nNone\n\nRemote-control command(s):\n[SENSe:]TRACking:LEVel ON | OFF", "Flags"={"OPC Wait"=FALSE, "Dont check status"=FALSE, "*WAI"=FALSE}, "Check Status Callback"=""}, {"Level"=3, "Descriptive Name"="WLAN Tracking Phase", "Class Only"=FALSE, "Data Type"=3, "Access"=2, "Identifier"="RSZVL_ATTR_WLAN_TRAC_PHAS", "Range Table"="", "Command"="SENS:TRAC:PHAS", "Read Callback"="", "Write Callback"="", "Range Callback"="", "Check Callback"="", "Rngtable Callback"="", "Coerce Callback"="", "User Callback"="", "Supported Models"="", "Instrument Options"="", "Repeated Capabilities"="", "Restricted Repeated Capabilities"="", "Help"="This attribute defines whether or not the measurement results should be compensated for phase.\n\nAvailable Repeated Capabilities:\nNone\n\nRemote-control command(s):\n[SENSe:]TRACking:PHASe ON | OFF", "Flags"={"OPC Wait"=FALSE, "Dont check status"=FALSE, "*WAI"=FALSE}, "Check Status Callback"=""}, {"Level"=3, "Descriptive Name"="WLAN Tracking Timing", "Class Only"=FALSE, "Data Type"=3, "Access"=2, "Identifier"="RSZVL_ATTR_WLAN_TRAC_TIME", "Range Table"="", "Command"="SENS:TRAC:TIME", "Read Callback"="", "Write Callback"="", "Range Callback"="", "Check Callback"="", "Rngtable Callback"="", "Coerce Callback"="", "User Callback"="", "Supported Models"="", "Instrument Options"="", "Repeated Capabilities"="", "Restricted Repeated Capabilities"="", "Help"="This attribute defines whether or not the measurement results should be compensated for time.\n\nAvailable Repeated Capabilities:\nNone\n\nRemote-control command(s):\n[SENSe:]TRACking:TIME ON | OFF", "Flags"={"OPC Wait"=FALSE, "Dont check status"=FALSE, "*WAI"=FALSE}, "Check Status Callback"=""}, {"Level"=1, "Descriptive Name"="B6 TV Trigger", "Class Only"=TRUE, "Data Type"=0, "Access"=0, "Identifier"="", "Range Table"="", "Command"="", "Read Callback"="", "Write Callback"="", "Range Callback"="", "Check Callback"="", "Rngtable Callback"="", "Coerce Callback"="", "User Callback"="", "Supported Models"="", "Instrument Options"="", "Repeated Capabilities"="", "Restricted Repeated Capabilities"="", "Help"="This class contains the attribute that configure option B6 - TV Trigger.\n\n(1) Trigger RF Power Level:\nThis attribute sets the level of the RF power trigger source.\n\n(2) TV and RFP Trigger Source:\nThis attribute selects the trigger source for the start of a sweep.\n\n(3) TV Trigger Free Run Mode:\nThis attribute activates or deactivates the free run trigger mode.\n\n(4) TV Trigger Vertical Signal:\nThis attribute activates triggering at the vertical sync signal.\n\n(5) TV Trigger Line System:\nThis attribute defines the line system in use (525 or 625 lines) with active TV trigger.\n\n(6) TV Trigger Horizontal Sync Signal:\nThis attribute triggering at the horizontal sync signal of the indicated line number.\n\n(7) TV Trigger Video Signal Polarity:\nThis attribute selects the polarity of the video sync signal.", "Flags"={"OPC Wait"=FALSE, "Dont check status"=FALSE, "*WAI"=FALSE}, "Check Status Callback"=""}, {"Level"=2, "Descriptive Name"="TV Trigger Source", "Class Only"=FALSE, "Data Type"=0, "Access"=2, "Identifier"="RSZVL_ATTR_TRIGGER_SOURCE_TV", "Range Table"="rszvl_rngTriggerSourceB6", "Command"="TRIG:SOUR", "Read Callback"="", "Write Callback"="", "Range Callback"="", "Check Callback"="", "Rngtable Callback"="", "Coerce Callback"="", "User Callback"="", "Supported Models"="", "Instrument Options"="", "Repeated Capabilities"="", "Restricted Repeated Capabilities"="", "Help"="This attribute selects the TV trigger source for the start of a sweep.\n\nAvailable Repeated Capabilities:\nNone\n\nRemote-control command(s):\nTRIGger<1|2>[:SEQuence]:SOURce TV", "Flags"={"OPC Wait"=FALSE, "Dont check status"=FALSE, "*WAI"=FALSE}, "Check Status Callback"=""}, {"Level"=2, "Descriptive Name"="TV Trigger Free Run Mode", "Class Only"=FALSE, "Data Type"=3, "Access"=2, "Identifier"="RSZVL_ATTR_TRIGGER_TV_VID_CONT", "Range Table"="", "Command"="TRIG:VID:CONT", "Read Callback"="", "Write Callback"="", "Range Callback"="", "Check Callback"="", "Rngtable Callback"="", "Coerce Callback"="", "User Callback"="", "Supported Models"="", "Instrument Options"="", "Repeated Capabilities"="", "Restricted Repeated Capabilities"="", "Help"="This attribute activates or deactivates the free run trigger mode.\n\nAvailable Repeated Capabilities:\nNone\n\nRemote-control command(s):\nTRIGger<1|2>[:SEQuence]:VIDeo:CONTinuous ON | OFF", "Flags"={"OPC Wait"=FALSE, "Dont check status"=FALSE, "*WAI"=FALSE}, "Check Status Callback"=""}, {"Level"=2, "Descriptive Name"="TV Trigger Vertical Signal", "Class Only"=FALSE, "Data Type"=0, "Access"=2, "Identifier"="RSZVL_ATTR_TRIGGER_TV_VERTICAL_SIGNAL", "Range Table"="rszvl_rngTriggerTVVertSig", "Command"="TRIG:VID:FIEL:SEL", "Read Callback"="", "Write Callback"="", "Range Callback"="", "Check Callback"="", "Rngtable Callback"="", "Coerce Callback"="", "User Callback"="", "Supported Models"="", "Instrument Options"="", "Repeated Capabilities"="", "Restricted Repeated Capabilities"="", "Help"="This attribute activates triggering at the vertical sync signal.\n\nAvailable Repeated Capabilities:\nNone\n\nRemote-control command(s):\nTRIGger<1|2>[:SEQuence]:VIDeo:FIELd:SELect ALL | ODD | EVEN", "Flags"={"OPC Wait"=FALSE, "Dont check status"=FALSE, "*WAI"=FALSE}, "Check Status Callback"=""}, {"Level"=2, "Descriptive Name"="TV Trigger Line System", "Class Only"=FALSE, "Data Type"=0, "Access"=2, "Identifier"="RSZVL_ATTR_TRIGGER_TV_LINE_SYSTEM", "Range Table"="rszvl_rngTriggerTVLineSystem", "Command"="TRIG:VID:FORM:LPFR", "Read Callback"="", "Write Callback"="", "Range Callback"="", "Check Callback"="", "Rngtable Callback"="", "Coerce Callback"="", "User Callback"="", "Supported Models"="", "Instrument Options"="", "Repeated Capabilities"="", "Restricted Repeated Capabilities"="", "Help"="This attribute defines the line system in use (525 or 625 lines) with active TV trigger.\n\nAvailable Repeated Capabilities:\nNone\n\nRemote-control command(s):\nTRIGger<1|2>[:SEQuence]:VIDeo:FORMat:LPFRame", "Flags"={"OPC Wait"=FALSE, "Dont check status"=FALSE, "*WAI"=FALSE}, "Check Status Callback"=""}, {"Level"=2, "Descriptive Name"="TV Trigger Horizontal Sync Signal", "Class Only"=FALSE, "Data Type"=0, "Access"=2, "Identifier"="RSZVL_ATTR_TRIGGER_TV_HORIZONTAL_SIGNAL", "Range Table"="", "Command"="TRIG:VID:LINE:NUMB", "Read Callback"="", "Write Callback"="", "Range Callback"="", "Check Callback"="", "Rngtable Callback"="", "Coerce Callback"="", "User Callback"="", "Supported Models"="", "Instrument Options"="", "Repeated Capabilities"="", "Restricted Repeated Capabilities"="", "Help"="This attribute triggering at the horizontal sync signal of the indicated line number.\n\nAvailable Repeated Capabilities:\nNone\n\nRemote-control command(s):\nTRIGger<1|2>[:SEQuence]:VIDeo:LINE:NUMBer", "Flags"={"OPC Wait"=FALSE, "Dont check status"=FALSE, "*WAI"=FALSE}, "Check Status Callback"=""}, {"Level"=2, "Descriptive Name"="TV Trigger Video Signal Polarity", "Class Only"=FALSE, "Data Type"=0, "Access"=2, "Identifier"="RSZVL_ATTR_TRIGGER_TV_VIDEO_POLARITY", "Range Table"="rszvl_rngPolarity", "Command"="TRIG:VID:SSIG:POL", "Read Callback"="", "Write Callback"="", "Range Callback"="", "Check Callback"="", "Rngtable Callback"="", "Coerce Callback"="", "User Callback"="", "Supported Models"="", "Instrument Options"="", "Repeated Capabilities"="", "Restricted Repeated Capabilities"="", "Help"="This attribute selects the polarity of the video sync signal.\n\nAvailable Repeated Capabilities:\nNone\n\nRemote-control command(s):\nTRIGger<1|2>[:SEQuence]:VIDeo:SSIGnal:POLarity", "Flags"={"OPC Wait"=FALSE, "Dont check status"=FALSE, "*WAI"=FALSE}, "Check Status Callback"=""}] {"Access" items=["Read Only", "Write Only", "Read/Write"]; "Data Type" items=["ViInt32", "ViReal64", "ViString", "ViBoolean", "None"]}
